vi "Get Control References.vi"(3 "error in":errorcluster, 5 "This vi":refnum<vi>) -> (0 "error out":errorcluster, 1 "Control Names":string[](array[string]), 2 "Controls[]":refnum<vi>[](array[refnum]))   [LabVIEW 2018]
doc: "Returns an array of control references and a string array of control label names, from the front panel of the calling VI.\n\nThis VI also accounts for tab controls within other tab controls."
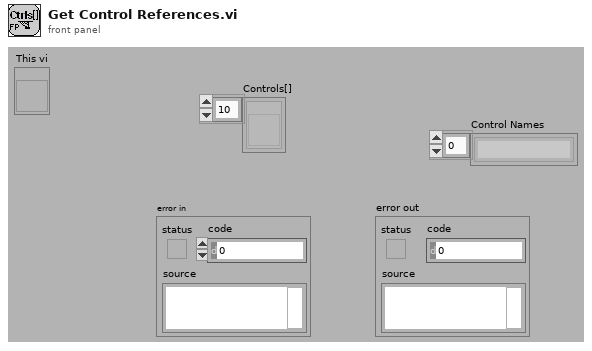
[diagram p1: front panel]
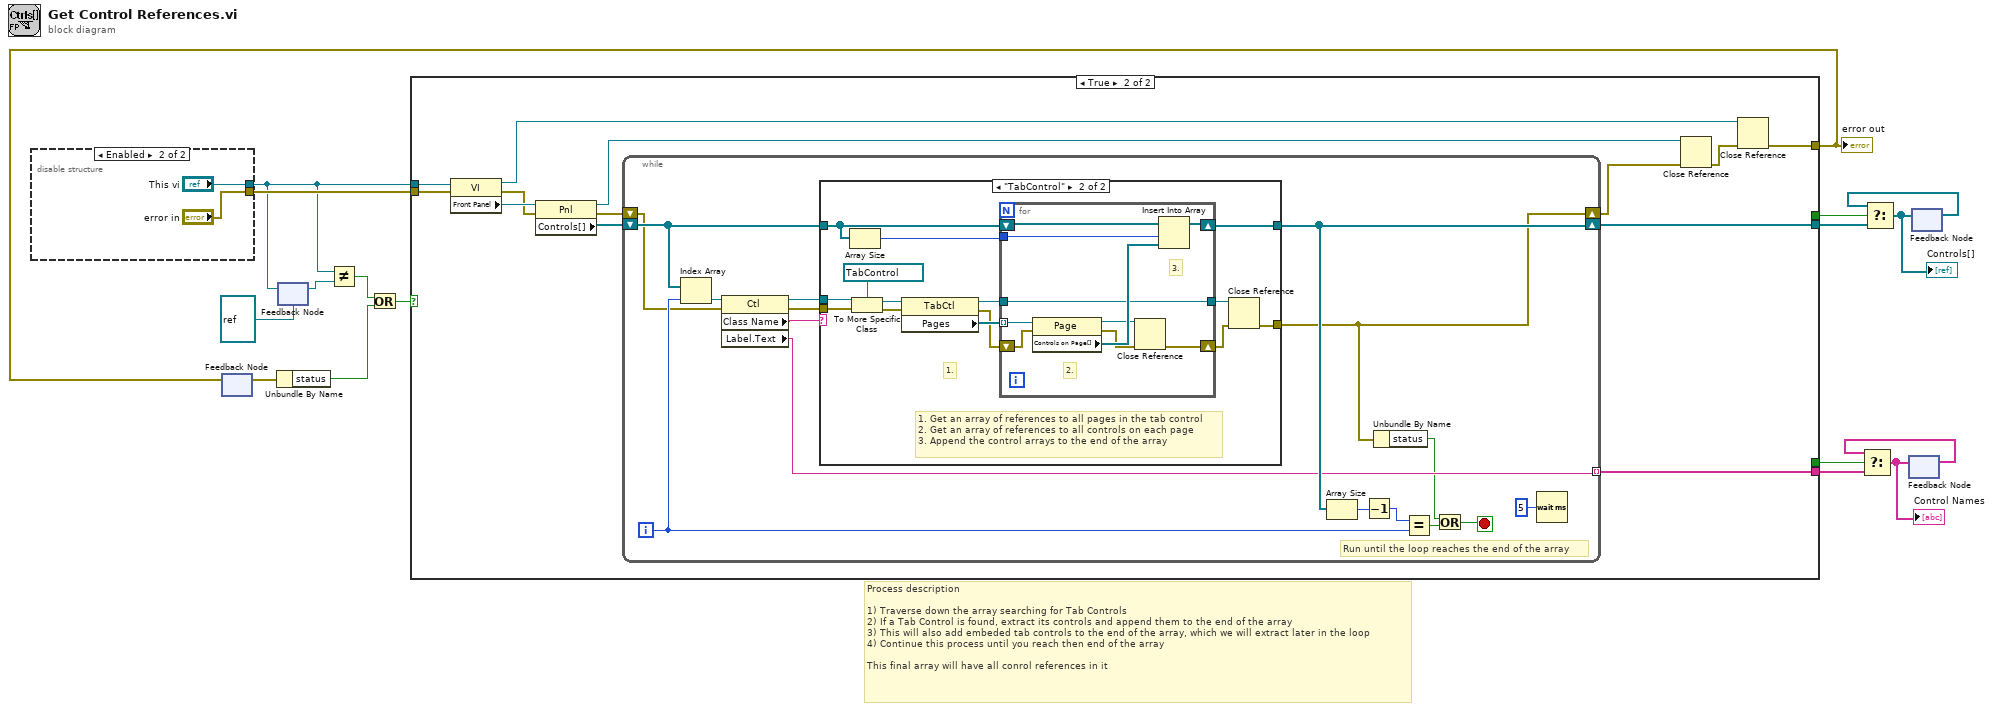
[diagram p0: block diagram]
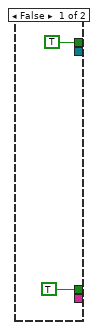
[diagram p2: hidden frame]
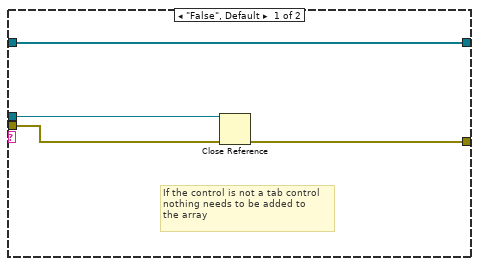
[diagram p3: hidden frame]
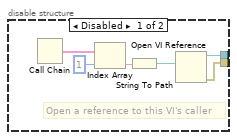
[diagram p4: hidden frame]
diagram:
  # "Process description\n\n1) Traverse down the array searching for Tab Controls\n2) If a Tab Control is found, extract its controls and append them to the end of the array\n3) This will also add embeded tab controls to the end of the array, which we will extract later in the loop\n4) Continue this process until you reach then end of the array\n\nThis final array will have all conrol references in it"
  n1 = disable-structure shown="Enabled" {
    disable-tunnel: [w19 "This vi"] -> w15
    disable-tunnel: [w18 "error in"] -> w17
    frame Disabled {
      # "Open a reference to this VI's caller"
      n2 = Call Chain() -> (call chain=w22:string[])
      n3 = Index Array(array=w22, index=1) -> (element=w21:string)
      n4 = String To Path(string=w21) -> (path=w20:path)
      n5 = Open VI Reference(vi path=w20) -> (vi reference=w19:refnum<vi>, error out=w18:errorcluster)  [unwired: 5 in]
    }
    frame Enabled {
    }
  }
  n6 = feedback #1() -> (w10:errorcluster)  [unwired: 1 in]
  n7 = Unbundle By Name(w10) -> ("status"=w9:bool)
  n8 = feedback #2(refnum<vi> refnum ("This vi")) -> (w16:refnum<vi>)
  n9 = feedback-in #2(w15) -> ()
  n10 = Not Equal?(x=w15, y=w16) -> (x != y?=w14:bool)
  n11 = Or(x=w14, y=w9) -> (x .or. y?=w13:bool)
  n12 = case shown="True" w13 {
    tunnel: [_ w40] -> w2
    tunnel: [_ w39] -> w6
    tunnel: w15 -> [_ w34]
    tunnel: w17 -> [_ w33]
    tunnel: [_ w28] -> w11
    tunnel: [TRUE ("s") _] -> w8
    tunnel: [TRUE ("s") _] -> w3
    frame False {
    }
    frame True {
      n13 = property class="VI"(reference=w34, error in=w33) -> (reference out=w32:refnum<vi>, error out=w36:errorcluster, "Front Panel"=w37:refnum<vi>)
      n14 = property class="Pnl"(reference=w37, error in=w36) -> (reference out=w31:refnum<vi>, error out=w35:errorcluster, "Controls[]"=w38:refnum<vi>[])
      n15 = while {
        shift-right: [w48] -> w39
        shift-left: w38 -> [w54]
        tunnel: [w45] -> w40 mode=indexing
        shift-right: [w44] -> w29
        shift-left: w35 -> [w47]
        i -> [w49]
        stop <- w42 stop-if-true
        # "Run until the loop reaches the end of the array"
        n16 = Index Array(array=w54, index=w49) -> (element=w50:refnum<vi>)
        n17 = property class="Ctl"(reference=w50, error in=w47) -> (reference out=w55:refnum<vi>, error out=w46:errorcluster, "Class Name"=w53:string, "Label.Text"=w45:string)
        n18 = case shown="\"TabControl\"" w53 {
          tunnel: w55 -> [w59 w74]
          tunnel: w54 -> [w60 w70]
          tunnel: [w60 w71] -> w48
          tunnel: w46 -> [w58 w67]
          tunnel: [w57 w63] -> w44
          frame "False", Default {
            # "If the control is not a tab control\nnothing needs to be added to\nthe array"
            n19 = Close Reference(reference=w59, error in (no error)=w58) -> (error out=w57:errorcluster)
          }
          frame "TabControl" {
            # "1. Get an array of references to all pages in the tab control\n2. Get an array of references to all controls on each page\n3. Append the control arrays to the end of the array"
            # "1."
            n20 = Array Size(array=w70) -> (size(s)=w68:i32)
            n21 = To More Specific Class(target class=refnum<vi> refnum ("Tab Control"), reference=w74, error in=w67) -> (specific class reference=w73:refnum<vi>, error out=w66:errorcluster)
            n22 = property class="TabCtl"(reference=w73, error in=w66) -> (reference out=w64:refnum<vi>, error out=w65:errorcluster, "Pages"=w72:refnum<vi>[])
            n23 = for {
              tunnel: w72 -> [w84] mode=indexing
              tunnel: w68 -> [w82]
              shift-right: [w83] -> w71
              shift-left: w70 -> [w81]
              tunnel: w64 -> [w78]
              tunnel: [w78] -> w62
              shift-right: [w75] -> w61
              shift-left: w65 -> [w79]
              # "3."
              # "2."
              n24 = property class="Page"(reference=w84, error in=w79) -> (reference out=w77:refnum<vi>, error out=w76:errorcluster, "Controls on Page[]"=w80:refnum<vi>[])
              n25 = Close Reference(reference=w77, error in (no error)=w76) -> (error out=w75:errorcluster)
              n26 = Insert Into Array(array=w81, index=w82, new element=w80) -> (w83:refnum<vi>[])
            }
            n27 = Close Reference(reference=w62, error in (no error)=w61) -> (error out=w63:errorcluster)
          }
        }
        n28 = Array Size(array=w48) -> (size(s)=w52:i32)
        n29 = Decrement(x=w52) -> (x-1=w51:i32)
        n30 = Unbundle By Name(w44) -> ("status"=w41:bool)
        n31 = Equal?(x=w51, y=w49) -> (x = y?=w43:bool)
        n32 = Or(x=w41, y=w43) -> (x .or. y?=w42:bool)
        n33 = Wait (ms)(milliseconds to wait=u32 5) -> ()  [unwired: 1 out]
      }
      n34 = Close Reference(reference=w31, error in (no error)=w29) -> (error out=w30:errorcluster)
      n35 = Close Reference(reference=w32, error in (no error)=w30) -> (error out=w28:errorcluster)
    }
  }
  "error out" <- w11
  n36 = feedback-in #1(w11) -> ()
  n37 = feedback #3() -> (w4:string[])  [unwired: 1 in]
  n38 = Select(t=w4, s=w3, f=w2) -> (s? t:f=w1:string[])
  "Control Names" <- w1
  n39 = feedback-in #3(w1) -> ()
  n40 = feedback #4() -> (w7:refnum<vi>[])  [unwired: 1 in]
  n41 = Select(t=w7, s=w8, f=w6) -> (s? t:f=w5:refnum<vi>[])
  "Controls[]" <- w5
  n42 = feedback-in #4(w5) -> ()
